vi "Review Modules Dialog.vi"(8 "error in":errorcluster, 11 "Potting Procedure in":refnum<class "Potting Procedure.lvclass">) -> (0 "error out":errorcluster, 2 "Canceled":bool, 3 "Potting Procedure out":refnum<class "Potting Procedure.lvclass">)   [LabVIEW 2011]
uses:
  Procedure Classes/Potting Procedure/Potting Procedure.lvclass
  Shared Components/Utils/Type Definitions/Fiducial with Source.ctl
  Shared Components/Vec3d Class/Vec3d Class.lvclass
  Procedure Classes/Potting Procedure/Type Definitions/Review Modules.ctl
  Procedure Classes/Potting Procedure/Type Definitions/Inspect Modules.ctl
  Shared Components/Utils/Type Definitions/Multi-Fiducial Image.ctl
  Shared Components/Utils/Type Definitions/Physical Image.ctl
  <vilib>/vision/Image Controls.llb/IMAQ Image.ctl
  Shared Components/Utils/Type Definitions/Fiducial Image.ctl
panel:
  in  "idx":i32
  out "idx_label":string="1/10"
  out "Current Module":cluster{"Chuck":i32, "Slot":i32}={"Chuck"=1, "Slot"=1}
  in  "Previous":bool
  in  "Next":bool
  in  "Tab Control":enum32{"Bond Pads", "TBM", "Address Pads & HV"}(tab)
  out "BBM-R":cluster{"X":dbl, "Y":dbl}[](graph)
  out "BBM-L":cluster{"X":dbl, "Y":dbl}[](graph)
  out "HDI-R":cluster{"X":dbl, "Y":dbl}[](graph)
  out "HDI-L":cluster{"X":dbl, "Y":dbl}[](graph)
  out "BBM BR":T1(plugin-control)
  out "BBM BL":T1(plugin-control)
  out "BBM TR":T1(plugin-control)
  out "BBM TL":T1(plugin-control)
  out "HDI BR":T1(plugin-control)
  out "HDI BL":T1(plugin-control)
  out "HDI TR":T1(plugin-control)
  out "HDI TL":T1(plugin-control)
  out "TBM-HDI":T1(plugin-control)
  out "TBM-TBM":T1(plugin-control)
  out "addr":T1(plugin-control) caption="Address Pads"
  out "HV-HDI":T1(plugin-control)
  out "HV-BBM":T1(plugin-control)
  in  "OK Button":bool
  in  "Cancel Button":bool
  # "Click on images to correct fiducial positions.\nAll error fiducials must be corrected before continuing."
  # "Pattern Recognition"
  # "Error"
  # "User Defined"
  # "Default"
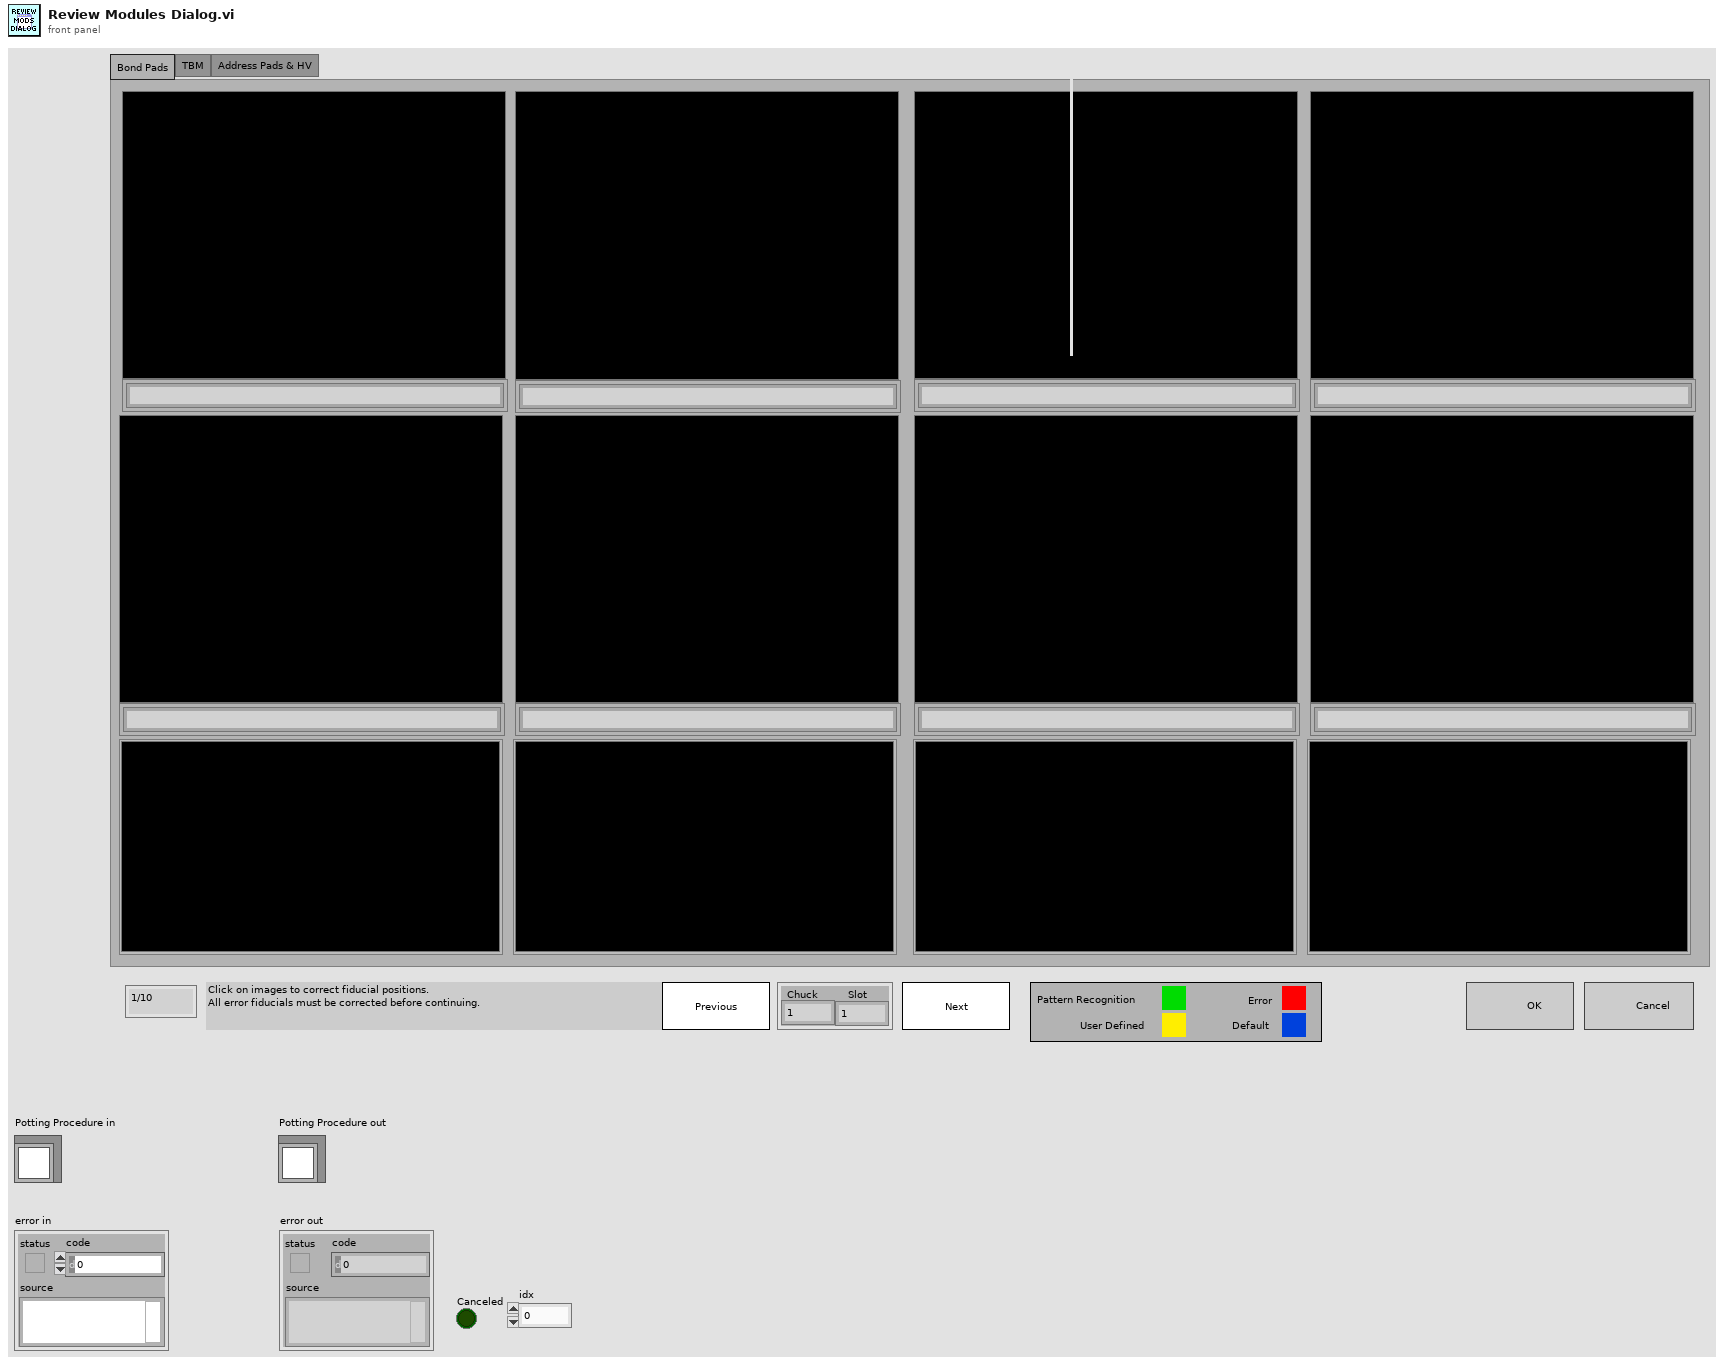
[diagram p1: front panel]
types:
  T1 = typedef "IMAQ Image.ctl" = refnum<image>
  T2 = typedef "Inspect Modules.ctl" = cluster{"Has Been Run?":bool, "Module Positions":cluster{"TBM-TBM":T3, "TBM-HDI":T3, "Address Pads":T3, "HDI Bond Pad References":T6[], "BBM Bond Pad References":T6[], "HV-HDI":T6, "HV-BBM":T6, "Chuck":i32, "Slot":i32}[]}
  T3 = typedef "Multi-Fiducial Image.ctl" = cluster{"Fiducial Image":T4, "Fiducials":cluster{"Selected Fiducial":T5, "fiducial name":string}[]}
  T4 = typedef "Physical Image.ctl" = cluster{"Image Position":refnum<class "Vec3d Class.lvclass">, "Image Reference":T1, "Field of View":cluster{"x(mm)":dbl, "y(mm)":dbl}}
  T5 = typedef "Fiducial with Source.ctl" = cluster{"Fiducial Image Coordinate":refnum<class "Vec3d Class.lvclass">, "Fiducial Source":enum16{"Pattern Recognition", "User", "Error", "Default"}}
  T6 = typedef "Fiducial Image.ctl" = cluster{"Fiducial Image":T4, "Selected Fiducial":T5, "fiducial name":string}
  T7 = cluster{"TBM-TBM":T3, "TBM-HDI":T3, "Address Pads":T3, "HDI Bond Pad References":T6[], "BBM Bond Pad References":T6[], "HV-HDI":T6, "HV-BBM":T6, "Chuck":i32, "Slot":i32}[]
  T8 = enum16{"Pattern Recognition", "User", "Error", "Default"}
  T9 = typedef "LVPoint32TypeDef.ctl" = cluster{"Horizontal":i32, "Vertical":i32}
  T10 = cluster{"TBM-TBM":T3, "TBM-HDI":T3, "Address Pads":T3, "HDI Bond Pad References":T6[], "BBM Bond Pad References":T6[], "HV-HDI":T6, "HV-BBM":T6, "Chuck":i32, "Slot":i32}
  T11 = cluster{"Selected Fiducial":T5, "fiducial name":string}[]
  T12 = cluster{"Selected Fiducial":T5, "fiducial name":string}
  T13 = typedef "eventvkey.ctl" = enum16{"ASCII", "Enter", "Return", "Shift", "Ctrl", "Alt", "Cmd", "Opt", "Caps", "NumLock", "Clear", "Break", "Up", "Down", "Left", "Right", "Insert", "Delete", "Home", "End", "PageUp", "PageDown", "Escape", "Help", "Pause", "ScrollLock", "F1", "F2", "F3", "F4", "F5", "F6", "F7", "F8", "F9", "F10", "F11", "F12", "F13", "F14", "F15", "F16", "F17", "F18", "F19", "F20", "F21", "F22", "F23", "F24", "Play", "VolumeUp", "VolumeDown", "Mute", "Two Byte Char"}
  T14 = typedef "Review Modules.ctl" = cluster{"Has Been Run?":bool}
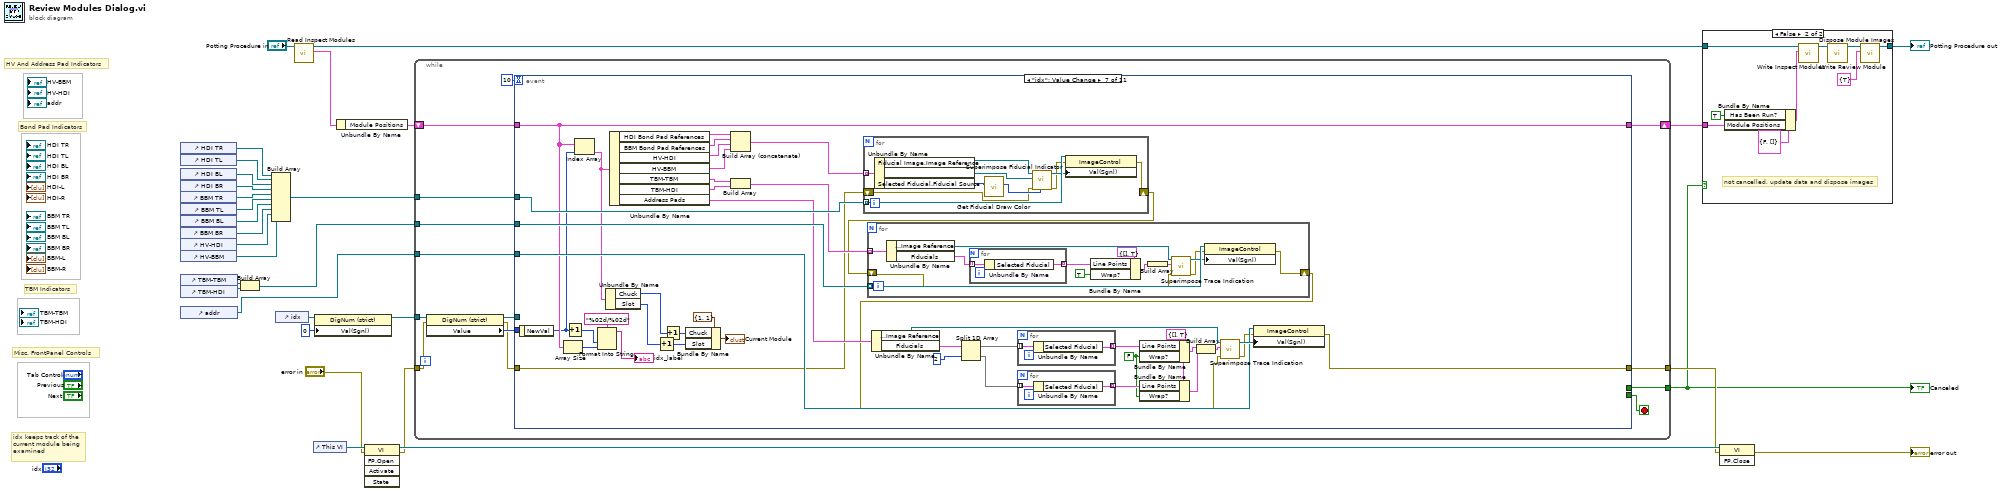
[diagram p0: block diagram]
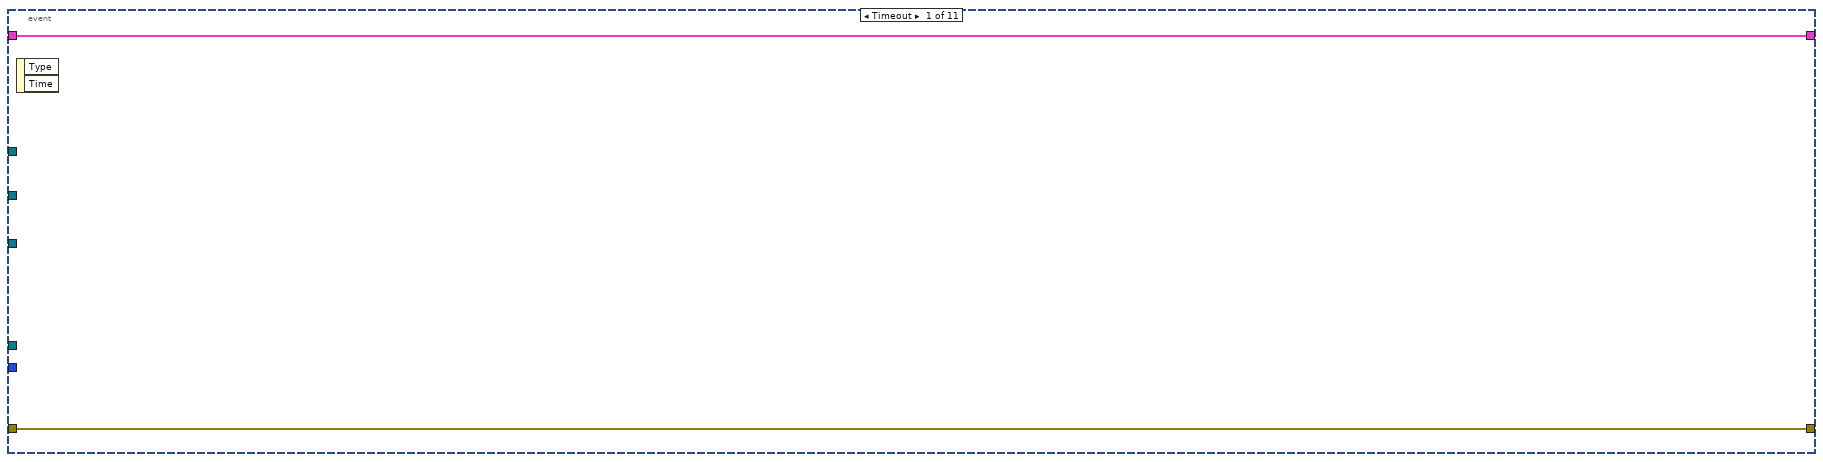
[diagram p3: hidden frame]
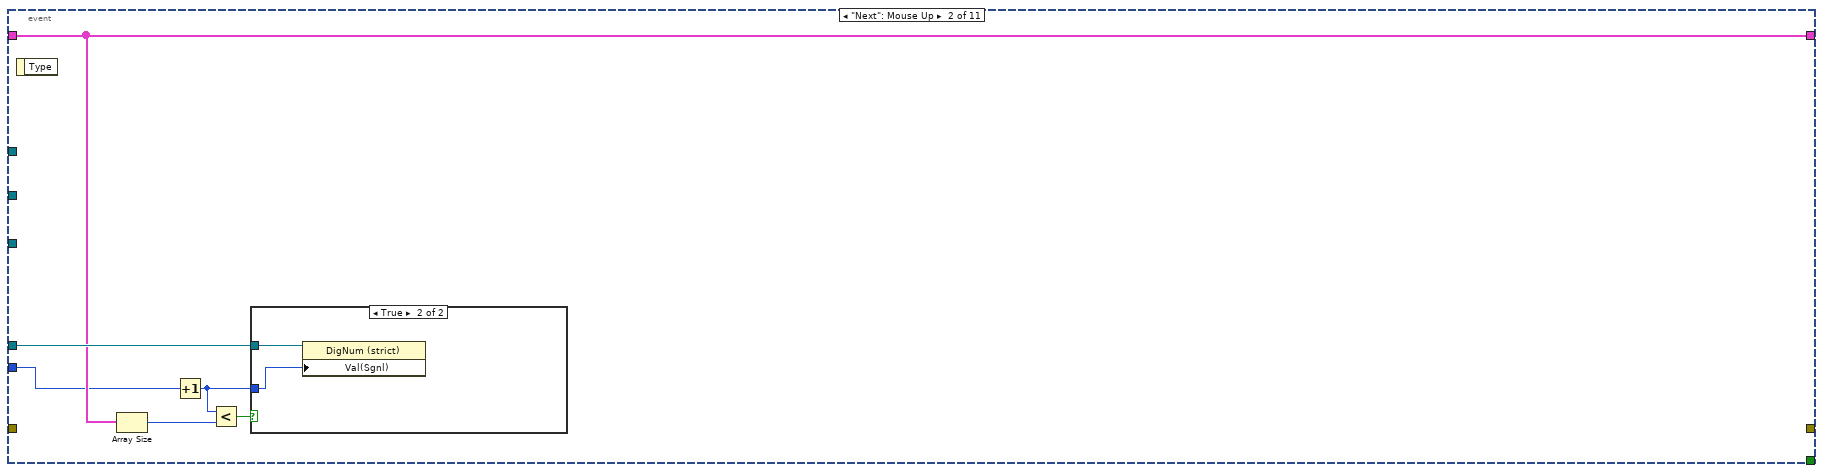
[diagram p4: hidden frame]
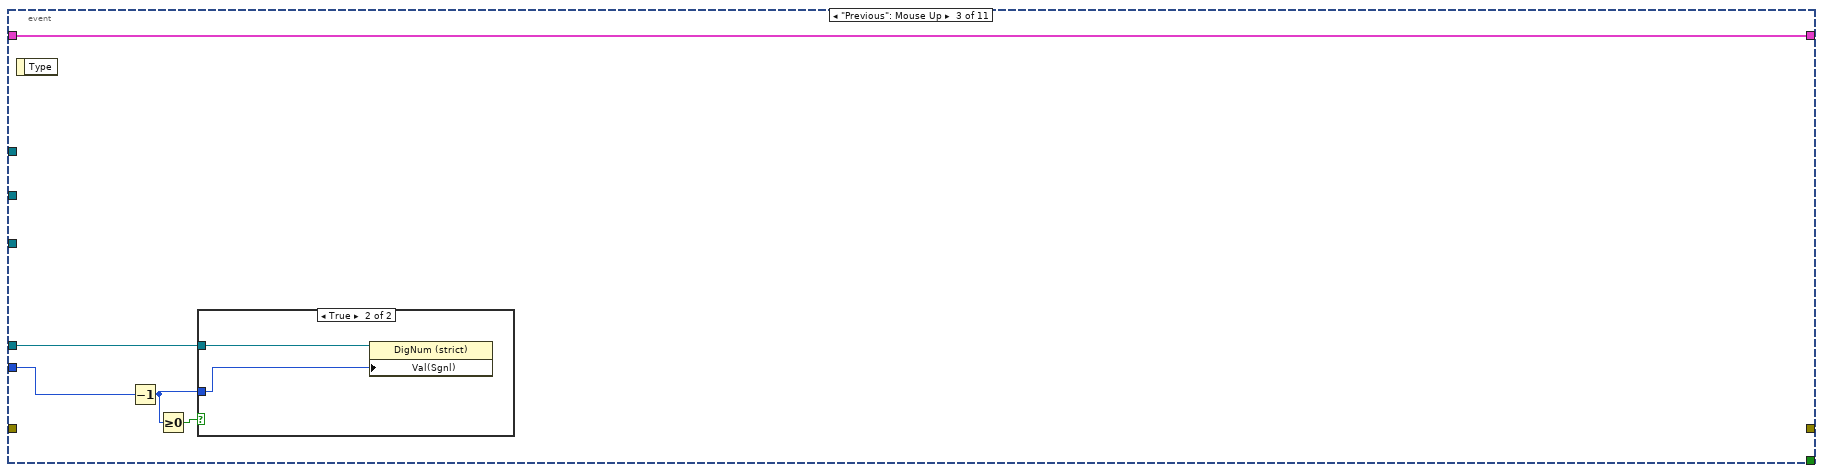
[diagram p6: hidden frame]
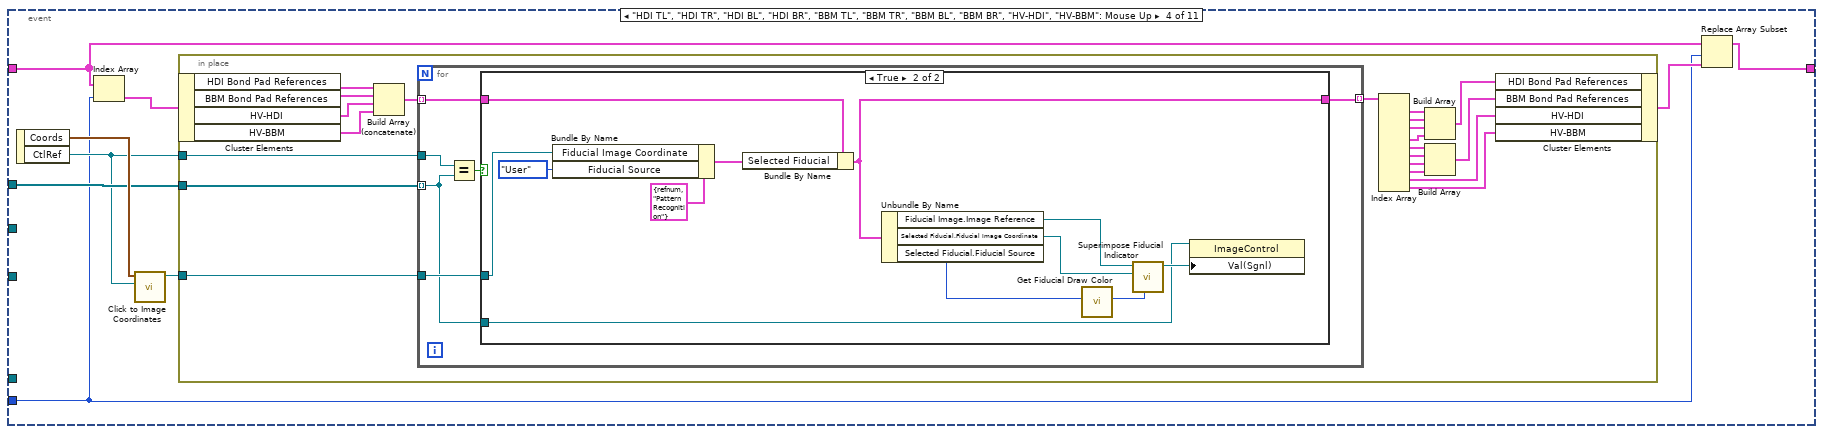
[diagram p8: hidden frame]
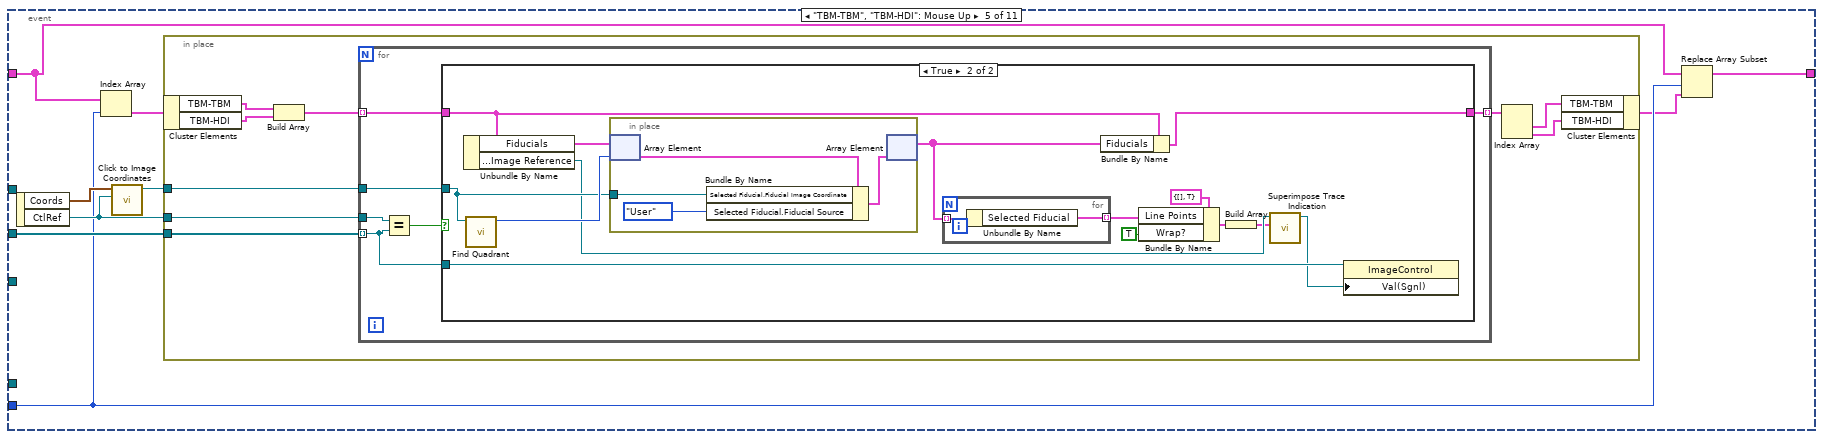
[diagram p10: hidden frame]
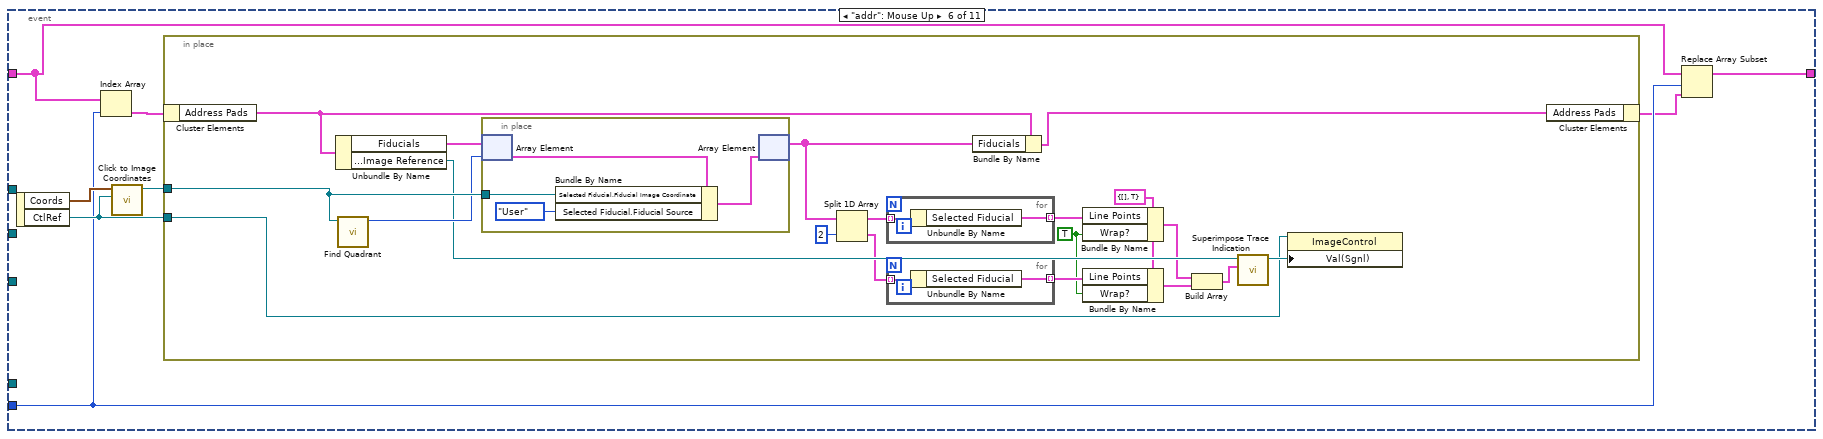
[diagram p12: hidden frame]
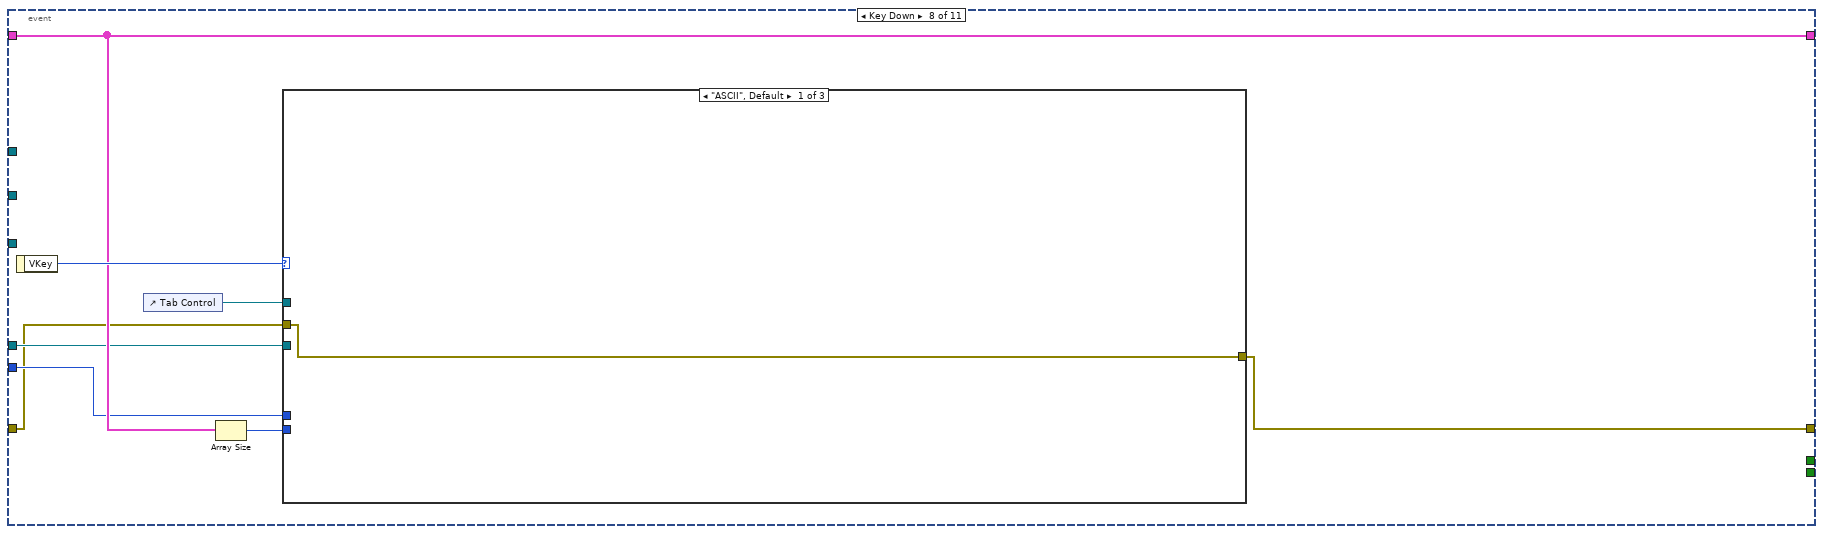
[diagram p13: hidden frame]
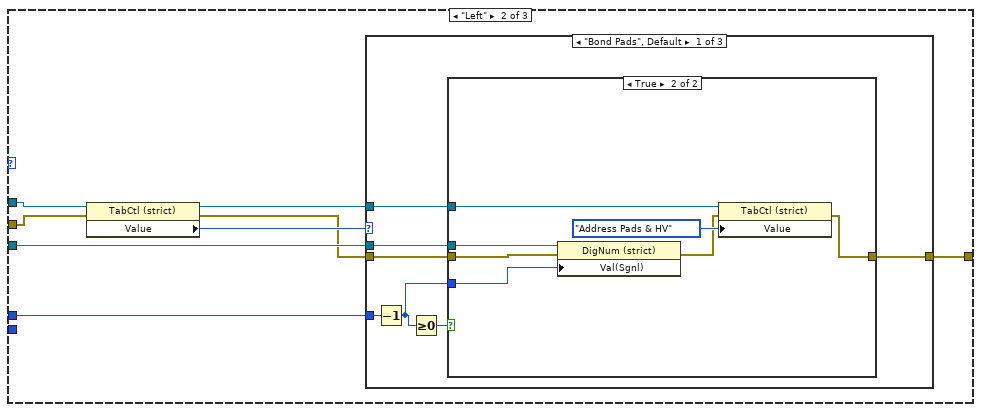
[diagram p14: hidden frame]
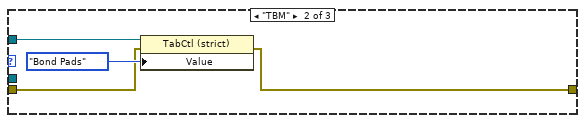
[diagram p16: hidden frame]
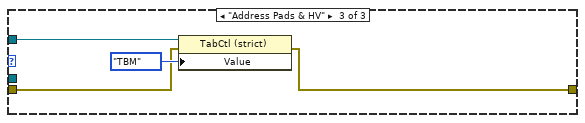
[diagram p17: hidden frame]
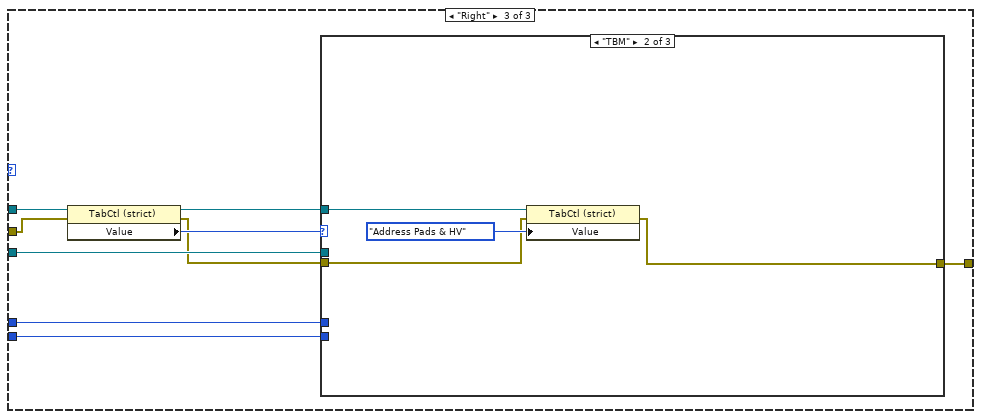
[diagram p18: hidden frame]
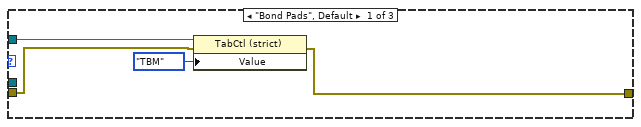
[diagram p19: hidden frame]
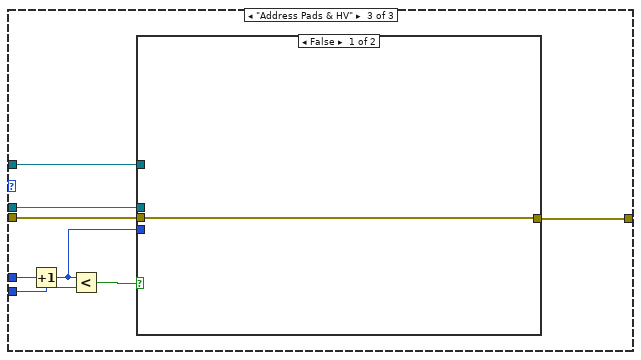
[diagram p20: hidden frame]
diagram:
  # "idx keeps track of the\ncurrent module being\nexamined"
  # "Misc. FrontPanel Controls"
  # "TBM Indicators"
  # "HV And Address Pad Indicators"
  # "Bond Pad Indicators"
  n1 = control-ref of="HDI TR"() -> (w22:refnum<vi>)
  n2 = control-ref of="HDI TL"() -> (w21:refnum<vi>)
  n3 = control-ref of="HDI BL"() -> (w20:refnum<vi>)
  n4 = control-ref of="HDI BR"() -> (w19:refnum<vi>)
  n5 = control-ref of="BBM TR"() -> (w18:refnum<vi>)
  n6 = control-ref of="BBM TL"() -> (w17:refnum<vi>)
  n7 = control-ref of="BBM BL"() -> (w16:refnum<vi>)
  n8 = control-ref of="BBM BR"() -> (w15:refnum<vi>)
  n9 = control-ref of="HV-HDI"() -> (w10:refnum<vi>)
  n10 = control-ref of="HV-BBM"() -> (w9:refnum<vi>)
  n11 = control-ref of="TBM-TBM"() -> (w13:refnum<vi>)
  n12 = control-ref of="TBM-HDI"() -> (w12:refnum<vi>)
  n13 = control-ref of="addr"() -> (w8:refnum<vi>)
  n14 = Build Array(w13, w12) -> (w11:refnum<vi>[])
  n15 = Build Array(w22, w21, w20, w19, w18, w17, w16, w15, w10, w9) -> (w14:refnum<vi>[])
  n16 = control-ref of="idx"() -> (w7:refnum<vi>)
  n17 = call-dynamic "Read Inspect Modules.vi"("Potting Procedure in"="Potting Procedure in") -> ("Inspect Modules"=w24:T2, "Potting Procedure out"=w2:refnum<class "Potting Procedure.lvclass">)  [unwired: 8 in, 1 out]
  n18 = control-ref of="This VI"() -> (w31:refnum<vi>)
  n19 = property class="DigNum (strict)"(reference=w7, "Val(Sgnl)"=0 ("Value (Signaling)")) -> (reference out=w6:refnum<vi>)  [unwired: 1 in, 1 out]
  n20 = Unbundle By Name(w24) -> ("Module Positions"=w23:T7)
  n21 = invoke class="VI" method="FP.Open"(reference=w31, error in="error in") -> (reference out=w30:refnum<vi>, error out=w27:errorcluster)  [unwired: 3 in, 3 out]
  n22 = while {
    tunnel: [w42] -> w4
    tunnel: w27 -> [w35]
    tunnel: [w43] -> w26
    shift-right: [w40] -> w3
    shift-left: w23 -> [w41]
    tunnel: w6 -> [w38]
    tunnel: w14 -> [w39]
    tunnel: w11 -> [w33]
    tunnel: w8 -> [w32]
    stop <- w44 stop-if-true
    n23 = property class="DigNum (strict)"(reference=w38, error in=w35) -> (reference out=w37:refnum<vi>, error out=w34:errorcluster, "Value"=w36:i32)
    n24 = event shown="[6] \"idx\": Value Change" {
      selector: _ -> [_ _ _ _ _ _ _ _ _ _ _]
      dyn-events: _ -> [_ _ _ _ _ _ _ _ _ _ _]
      timeout: 10 -> [_ _ _ _ _ _ _ _ _ _ _]
      tunnel: [_ _ _ _ _ _ _ _ w338 w340 _] -> w44
      tunnel: [w47 _ _ _ _ _ w205 w264 w339 w342 w345] -> w43
      tunnel: w34 -> [w47 _ _ _ _ _ w209 w265 w339 w342 w345]
      tunnel: [_ _ _ _ _ _ _ _ w338 _ _] -> w42
      tunnel: w41 -> [w46 w49 w57 w66 w113 w158 w195 w269 w337 w341 w344]
      tunnel: [w46 w49 w57 w63 w112 w157 w195 w269 w337 w341 w344] -> w40
      tunnel: w37 -> [_ w51 w58 _ _ _ _ w266 _ _ _]
      tunnel: w39 -> [_ _ _ w69 _ _ w227 _ _ _ _]
      tunnel: w36 -> [_ w48 w56 w64 w115 w160 _ w267 _ _ _]
      tunnel: w33 -> [_ _ _ _ w118 _ w225 _ _ _ _]
      tunnel: w32 -> [_ _ _ _ _ _ w218 _ _ _ _]
      event Timeout {
        n25 = event-data() -> ()  [unwired: 1 in, 2 out]
      }
      event "Next": Mouse Up {
        n26 = event-data() -> ()  [unwired: 1 in, 1 out]
        n27 = Array Size(array=w49) -> (size(s)=w50:i32)
        n28 = Increment(x=w48) -> (x+1=w52:i32)
        n29 = Less?(x=w52, y=w50) -> (x < y?=w53:bool)
        n30 = case shown="True" w53 {
          tunnel: w52 -> [_ w54]
          tunnel: w51 -> [_ w55]
          frame False {
          }
          frame True {
            n31 = property class="DigNum (strict)"(reference=w55, "Val(Sgnl)"=w54) -> ()  [unwired: 1 in, 2 out]
          }
        }
      }
      event "Previous": Mouse Up {
        n32 = event-data() -> ()  [unwired: 1 in, 1 out]
        n33 = Decrement(x=w56) -> (x-1=w59:i32)
        n34 = Greater Or Equal To 0?(x=w59) -> (x >= 0?=w60:bool)
        n35 = case shown="True" w60 {
          tunnel: w59 -> [_ w61]
          tunnel: w58 -> [_ w62]
          frame False {
          }
          frame True {
            n36 = property class="DigNum (strict)"(reference=w62, "Val(Sgnl)"=w61) -> ()  [unwired: 1 in, 2 out]
          }
        }
      }
      event "HDI TL", "HDI TR", "HDI BL", "HDI BR", "BBM TL", "BBM TR", "BBM BL", "BBM BR", "HV-HDI", "HV-BBM": Mouse Up {
        n37 = event-data() -> ("Coords"=w71:T9, "CtlRef"=w68:refnum<vi>)  [unwired: 1 in]
        n38 = Index Array(array=w66, index=w64) -> (element=w67:T10)
        n39 = call "Click to Image Coordinates.vi"("Display Reference"=w68, "Coords"=w71) -> ("Image Coordinates"=w70:refnum<class "Vec3d Class.lvclass">)  [unwired: 8 in, 1 out]
        n40 = in-place {
          in-place-border: w70 -> [w91]
          in-place-border: w69 -> [w90]
          in-place-border: w68 -> [w89]
          n41 = in-place-cluster #1(w67) -> ("HDI Bond Pad References"=w88:T6[], "BBM Bond Pad References"=w87:T6[], "HV-HDI"=w86:T6, "HV-BBM"=w85:T6)
          n42 = Build Array (concatenate)(w88, w87, w86, w85) -> (w92:T6[])
          n43 = for {
            tunnel: w92 -> [w95] mode=indexing
            tunnel: w91 -> [w96]
            tunnel: w90 -> [w94] mode=indexing
            tunnel: w89 -> [w98]
            tunnel: [w93] -> w84 mode=indexing
            n44 = Equal?(x=w98, y=w94) -> (x = y?=w97:bool)
            n45 = case shown="True" w97 {
              tunnel: w96 -> [_ w109]
              tunnel: w95 -> [w99 w111]
              tunnel: [w99 w106] -> w93
              tunnel: w94 -> [_ w102]
              frame False {
              }
              frame True {
                n46 = Bundle By Name(cluster=T5 {"Fiducial Image Coordinate"=refnum, "Fiducial Source"=enum."Pattern Recognition"} ("Selected Fiducial"), "Fiducial Image Coordinate"=w109, "Fiducial Source"=T8."User") -> (w107:T5)
                n47 = Bundle By Name(cluster=w111, "Selected Fiducial"=w107) -> (w106:T6)
                n48 = Unbundle By Name(w106) -> ("Fiducial Image.Image Reference"=w103:T1, "Selected Fiducial.Fiducial Image Coordinate"=w104:refnum<class "Vec3d Class.lvclass">, "Selected Fiducial.Fiducial Source"=w101:T8)
                n49 = call "Get Fiducial Draw Color.vi"("Fiducial Source"=w101) -> ("Grid Line Color"=w100:u32)  [unwired: 10 in]
                n50 = call "Superimpose Fiducial Indicator.vi"("Marker Color"=w100, "Fiducial Image Coordinates"=w104, "Image In"=w103) -> ("Image Out"=w105:T1)  [unwired: 7 in, 1 out]
                n51 = property class="ImageControl"(reference=w102, "Val(Sgnl)"=w105) -> ()  [unwired: 1 in, 2 out]
              }
            }
          }
          n52 = Index Array(array=w84) -> (element #1=w83:T6, element #2=w82:T6, element #3=w81:T6, element #4=w80:T6, element #5=w78:T6, element #6=w77:T6, element #7=w76:T6, element #8=w75:T6, element #9=w73:T6, element #10=w72:T6)  [unwired: 10 in]
          n53 = Build Array(w83, w82, w81, w80) -> (w79:T6[])
          n54 = Build Array(w78, w77, w76, w75) -> (w74:T6[])
          n55 = in-place-cluster #1("HDI Bond Pad References"=w79, "BBM Bond Pad References"=w74, "HV-HDI"=w73, "HV-BBM"=w72) -> (w65:T10)
        }
        n56 = Replace Array Subset(array=w66, new element=w65, index=w64) -> (w63:T7)
      }
      event "TBM-TBM", "TBM-HDI": Mouse Up {
        n57 = event-data() -> ("Coords"=w120:T9, "CtlRef"=w119:refnum<vi>)  [unwired: 1 in]
        n58 = Index Array(array=w113, index=w115) -> (element=w116:T10)
        n59 = call "Click to Image Coordinates.vi"("Display Reference"=w119, "Coords"=w120) -> ("Image Coordinates"=w117:refnum<class "Vec3d Class.lvclass">)  [unwired: 8 in, 1 out]
        n60 = in-place {
          in-place-border: w119 -> [w128]
          in-place-border: w118 -> [w127]
          in-place-border: w117 -> [w126]
          n61 = in-place-cluster #2(w116) -> ("TBM-TBM"=w125:T3, "TBM-HDI"=w124:T3)
          n62 = Build Array(w125, w124) -> (w129:T3[])
          n63 = for {
            tunnel: w129 -> [w133] mode=indexing
            tunnel: w128 -> [w135]
            tunnel: w127 -> [w131] mode=indexing
            tunnel: w126 -> [w132]
            tunnel: [w130] -> w123 mode=indexing
            n64 = Equal?(x=w135, y=w131) -> (x = y?=w134:bool)
            n65 = case shown="True" w134 {
              tunnel: w133 -> [w136 w147]
              tunnel: w132 -> [_ w148]
              tunnel: [w136 w146] -> w130
              tunnel: w131 -> [_ w138]
              frame False {
              }
              frame True {
                n66 = Unbundle By Name(w147) -> ("Fiducials"=w150:T11, "Fiducial Image.Image Reference"=w142:T1)
                n67 = call "Find Quadrant.vi"("Image Coordinate"=w148) -> ("Quadrant"=w149:i32)  [unwired: 10 in]
                n68 = in-place {
                  in-place-border: w148 -> [w154]
                  n69 = in-place-array #3(w150, w149) -> (w156:T12)
                  n70 = Bundle By Name(cluster=w156, "Selected Fiducial.Fiducial Image Coordinate"=w154, "Selected Fiducial.Fiducial Source"=T8."User") -> (w155:T12)
                  n71 = in-place-array #3(w155) -> (w145:T11)  [unwired: 1 out]
                }
                n72 = for {
                  tunnel: w145 -> [w152] mode=indexing
                  tunnel: [w151] -> w141 mode=indexing
                  n73 = Unbundle By Name(w152) -> ("Selected Fiducial"=w151:T5)
                }
                n74 = Bundle By Name(cluster=w147, "Fiducials"=w145) -> (w146:T3)
                n75 = Bundle By Name(cluster=cluster{"Line Points":T5[], "Wrap?":bool} {"Line Points"=[], "Wrap?"=TRUE} ("Line Group"), "Line Points"=w141, "Wrap?"=TRUE) -> (w144:cluster{"Line Points":T5[], "Wrap?":bool})
                n76 = Build Array(w144) -> (w139:cluster{"Line Points":T5[], "Wrap?":bool}[])
                n77 = call "Superimpose Trace Indication.vi"("Line Data"=w139, "Image In"=w142) -> ("Image Out"=w137:T1)  [unwired: 8 in, 1 out]
                n78 = property class="ImageControl"(reference=w138, "Val(Sgnl)"=w137) -> ()  [unwired: 1 in, 2 out]
              }
            }
          }
          n79 = Index Array(array=w123) -> (element #1=w122:T3, element #2=w121:T3)  [unwired: 2 in]
          n80 = in-place-cluster #2("TBM-TBM"=w122, "TBM-HDI"=w121) -> (w114:T10)
        }
        n81 = Replace Array Subset(array=w113, new element=w114, index=w115) -> (w112:T7)
      }
      event "addr": Mouse Up {
        n82 = event-data() -> ("Coords"=w164:T9, "CtlRef"=w163:refnum<vi>)  [unwired: 1 in]
        n83 = Index Array(array=w158, index=w160) -> (element=w161:T10)
        n84 = call "Click to Image Coordinates.vi"("Display Reference"=w163, "Coords"=w164) -> ("Image Coordinates"=w162:refnum<class "Vec3d Class.lvclass">)  [unwired: 8 in, 1 out]
        n85 = in-place {
          in-place-border: w163 -> [w174]
          in-place-border: w162 -> [w183]
          w165 = cluster{"Line Points":T5[], "Wrap?":bool} {"Line Points"=[], "Wrap?"=TRUE} ("Line Group")
          w168 = TRUE ("Wrap?")
          n86 = in-place-cluster #4(w161) -> ("Address Pads"=w181:T3)
          n87 = Unbundle By Name(w181) -> ("Fiducials"=w180:T11, "Fiducial Image.Image Reference"=w178:T1)
          n88 = call "Find Quadrant.vi"("Image Coordinate"=w183) -> ("Quadrant"=w179:i32)  [unwired: 10 in]
          n89 = in-place {
            in-place-border: w183 -> [w189]
            n90 = in-place-array #5(w180, w179) -> (w191:T12)
            n91 = Bundle By Name(cluster=w191, "Selected Fiducial.Fiducial Image Coordinate"=w189, "Selected Fiducial.Fiducial Source"=T8."User") -> (w190:T12)
            n92 = in-place-array #5(w190) -> (w172:T11)  [unwired: 1 out]
          }
          n93 = Split 1D Array(array=w172, index=2) -> (first subarray=w171:T11, second subarray=w170:T11)
          n94 = for {
            tunnel: [w186] -> _ mode=indexing
            tunnel: [w187] -> w177 mode=indexing
            tunnel: w171 -> [w186] mode=indexing
            n95 = Unbundle By Name(w186) -> ("Selected Fiducial"=w187:T5)
          }
          n96 = for {
            tunnel: w170 -> [w185] mode=indexing
            tunnel: [w184] -> w173 mode=indexing
            n97 = Unbundle By Name(w185) -> ("Selected Fiducial"=w184:T5)
          }
          n98 = Bundle By Name(cluster=w181, "Fiducials"=w172) -> (w182:T3)
          n99 = Bundle By Name(cluster=w165, "Line Points"=w177, "Wrap?"=w168) -> (w167:cluster{"Line Points":T5[], "Wrap?":bool})
          n100 = Bundle By Name(cluster=w165, "Line Points"=w173, "Wrap?"=w168) -> (w166:cluster{"Line Points":T5[], "Wrap?":bool})
          n101 = Build Array(w167, w166) -> (w176:cluster{"Line Points":T5[], "Wrap?":bool}[])
          n102 = call "Superimpose Trace Indication.vi"("Line Data"=w176, "Image In"=w178) -> ("Image Out"=w175:T1)  [unwired: 8 in, 1 out]
          n103 = property class="ImageControl"(reference=w174, "Val(Sgnl)"=w175) -> ()  [unwired: 1 in, 2 out]
          n104 = in-place-cluster #4("Address Pads"=w182) -> (w159:T10)
        }
        n105 = Replace Array Subset(array=w158, new element=w159, index=w160) -> (w157:T7)
      }
      event "idx": Value Change {
        w212 = FALSE ("Wrap?")
        w211 = cluster{"Line Points":T5[], "Wrap?":bool} {"Line Points"=[], "Wrap?"=TRUE} ("Line Group")
        n106 = event-data() -> ("NewVal"=w194:i32)  [unwired: 1 in]
        n107 = Array Size(array=w195) -> (size(s)=w201:i32)
        n108 = Increment(x=w194) -> (x+1=w202:i32)
        n109 = Index Array(array=w195, index=w194) -> (element=w196:T10)
        n110 = Format Into String(format string="%02d/%02d", w202, w201) -> (resulting string=→"idx_label":string)  [unwired: 2 in, 1 out]
        n111 = Unbundle By Name(w196) -> ("Chuck"=w193:i32, "Slot"=w192:i32)
        n112 = Unbundle By Name(w196) -> ("HDI Bond Pad References"=w234:T6[], "BBM Bond Pad References"=w233:T6[], "HV-HDI"=w232:T6, "HV-BBM"=w231:T6, "TBM-TBM"=w230:T3, "TBM-HDI"=w229:T3, "Address Pads"=w219:T3)
        n113 = Increment(x=w192) -> (x+1=w200:i32)
        n114 = Increment(x=w193) -> (x+1=w199:i32)
        n115 = Bundle By Name(cluster=cluster{"Chuck":i32, "Slot":i32} {"Chuck"=1, "Slot"=1} ("Current Module"), "Chuck"=w199, "Slot"=w200) -> (→"Current Module":cluster{"Chuck":i32, "Slot":i32})
        n116 = Build Array (concatenate)(w234, w233, w232, w231) -> (w228:T6[])
        n117 = Build Array(w230, w229) -> (w226:T3[])
        n118 = for {
          tunnel: w227 -> [w258] mode=indexing
          tunnel: w228 -> [w263] mode=indexing
          shift-right: [w254] -> w208
          shift-left: w209 -> [w256]
          n119 = Unbundle By Name(w263) -> ("Fiducial Image.Image Reference"=w262:T1, "Selected Fiducial.Fiducial Image Coordinate"=w261:refnum<class "Vec3d Class.lvclass">, "Selected Fiducial.Fiducial Source"=w260:T8)
          n120 = call "Get Fiducial Draw Color.vi"("Fiducial Source"=w260) -> ("Grid Line Color"=w259:u32)  [unwired: 10 in]
          n121 = call "Superimpose Fiducial Indicator.vi"("Marker Color"=w259, "error in"=w256, "Fiducial Image Coordinates"=w261, "Image In"=w262) -> ("error out"=w255:errorcluster, "Image Out"=w257:T1)  [unwired: 6 in]
          n122 = property class="ImageControl"(reference=w258, error in=w255, "Val(Sgnl)"=w257) -> (error out=w254:errorcluster)  [unwired: 1 out]
        }
        n123 = for {
          tunnel: w225 -> [w249] mode=indexing
          tunnel: w226 -> [w251] mode=indexing
          shift-right: [w239] -> w207
          shift-left: w208 -> [w241]
          n124 = Unbundle By Name(w251) -> ("Fiducial Image.Image Reference"=w250:T1, "Fiducials"=w247:T11)
          n125 = for {
            tunnel: w247 -> [w253] mode=indexing
            tunnel: [w252] -> w245 mode=indexing
            n126 = Unbundle By Name(w253) -> ("Selected Fiducial"=w252:T5)
          }
          n127 = Bundle By Name(cluster=cluster{"Line Points":T5[], "Wrap?":bool} {"Line Points"=[], "Wrap?"=TRUE} ("Line Group"), "Line Points"=w245, "Wrap?"=TRUE) -> (w243:cluster{"Line Points":T5[], "Wrap?":bool})
          n128 = Build Array(w243) -> (w242:cluster{"Line Points":T5[], "Wrap?":bool}[])
          n129 = call "Superimpose Trace Indication.vi"("error in"=w241, "Line Data"=w242, "Image In"=w250) -> ("error out"=w240:errorcluster, "Image Out"=w248:T1)  [unwired: 7 in]
          n130 = property class="ImageControl"(reference=w249, error in=w240, "Val(Sgnl)"=w248) -> (error out=w239:errorcluster)  [unwired: 1 out]
        }
        n131 = Unbundle By Name(w219) -> ("Fiducial Image.Image Reference"=w224:T1, "Fiducials"=w217:T11)
        n132 = Split 1D Array(array=w217, index=2) -> (first subarray=w215:T11, second subarray=w214:T11)
        n133 = for {
          tunnel: w215 -> [w238] mode=indexing
          tunnel: [w237] -> w222 mode=indexing
          n134 = Unbundle By Name(w238) -> ("Selected Fiducial"=w237:T5)
        }
        n135 = for {
          tunnel: w214 -> [w236] mode=indexing
          tunnel: [w235] -> w213 mode=indexing
          n136 = Unbundle By Name(w236) -> ("Selected Fiducial"=w235:T5)
        }
        n137 = Bundle By Name(cluster=w211, "Line Points"=w222, "Wrap?"=w212) -> (w221:cluster{"Line Points":T5[], "Wrap?":bool})
        n138 = Bundle By Name(cluster=w211, "Line Points"=w213, "Wrap?"=w212) -> (w210:cluster{"Line Points":T5[], "Wrap?":bool})
        n139 = Build Array(w221, w210) -> (w220:cluster{"Line Points":T5[], "Wrap?":bool}[])
        n140 = call "Superimpose Trace Indication.vi"("error in"=w207, "Line Data"=w220, "Image In"=w224) -> ("error out"=w206:errorcluster, "Image Out"=w223:T1)  [unwired: 7 in]
        n141 = property class="ImageControl"(reference=w218, error in=w206, "Val(Sgnl)"=w223) -> (error out=w205:errorcluster)  [unwired: 1 out]
      }
      event Key Down {
        n142 = event-data() -> ("VKey"=w271:T13)  [unwired: 1 in]
        n143 = control-ref of="Tab Control"() -> (w270:refnum<vi>)
        n144 = Array Size(array=w269) -> (size(s)=w268:i32)
        n145 = case shown="\"ASCII\", Default" w271 {
          tunnel: w270 -> [_ w276 w312]
          tunnel: w268 -> [_ _ w308]
          tunnel: w267 -> [_ w277 w307]
          tunnel: w266 -> [_ w278 w309]
          tunnel: w265 -> [w272 w275 w306]
          tunnel: [w272 w273 w304] -> w264
          frame "ASCII", Default {
          }
          frame "Left" {
            n146 = property class="TabCtl (strict)"(reference=w276, error in=w275) -> (reference out=w279:refnum<vi>, error out=w274:errorcluster, "Value"=w280:enum32{"Bond Pads", "TBM", "Address Pads & HV"})
            n147 = case shown="\"Bond Pads\", Default" w280 {
              tunnel: w279 -> [w287 w299 w302]
              tunnel: w278 -> [w286 _ _]
              tunnel: w277 -> [w285 _ _]
              tunnel: w274 -> [w282 w297 w301]
              tunnel: [w281 w296 w300] -> w273
              frame "Bond Pads", Default {
                n148 = Decrement(x=w285) -> (x-1=w283:i32)
                n149 = Greater Or Equal To 0?(x=w283) -> (x >= 0?=w284:bool)
                n150 = case shown="True" w284 {
                  tunnel: w286 -> [_ w295]
                  tunnel: w287 -> [_ w294]
                  tunnel: w283 -> [_ w292]
                  tunnel: w282 -> [w288 w291]
                  tunnel: [w288 w289] -> w281
                  frame False {
                  }
                  frame True {
                    n151 = property class="DigNum (strict)"(reference=w295, error in=w291, "Val(Sgnl)"=w292) -> (error out=w290:errorcluster)  [unwired: 1 out]
                    n152 = property class="TabCtl (strict)"(reference=w294, error in=w290, "Value"=enum32{"Bond Pads", "TBM", "Address Pads & HV"}."Address Pads & HV") -> (error out=w289:errorcluster)  [unwired: 1 out]
                  }
                }
              }
              frame "TBM" {
                n153 = property class="TabCtl (strict)"(reference=w299, error in=w297, "Value"=enum32{"Bond Pads", "TBM", "Address Pads & HV"}."Bond Pads") -> (error out=w296:errorcluster)  [unwired: 1 out]
              }
              frame "Address Pads & HV" {
                n154 = property class="TabCtl (strict)"(reference=w302, error in=w301, "Value"=enum32{"Bond Pads", "TBM", "Address Pads & HV"}."TBM") -> (error out=w300:errorcluster)  [unwired: 1 out]
              }
            }
          }
          frame "Right" {
            n155 = property class="TabCtl (strict)"(reference=w312, error in=w306) -> (reference out=w310:refnum<vi>, error out=w305:errorcluster, "Value"=w311:enum32{"Bond Pads", "TBM", "Address Pads & HV"})
            n156 = case shown="\"TBM\"" w311 {
              tunnel: w310 -> [w315 w320 w323]
              tunnel: w309 -> [_ _ w325]
              tunnel: w308 -> [_ _ w327]
              tunnel: w307 -> [_ _ w328]
              tunnel: w305 -> [w314 w318 w322]
              tunnel: [w313 w317 w321] -> w304
              frame "Bond Pads", Default {
                n157 = property class="TabCtl (strict)"(reference=w315, error in=w314, "Value"=enum32{"Bond Pads", "TBM", "Address Pads & HV"}."TBM") -> (error out=w313:errorcluster)  [unwired: 1 out]
              }
              frame "TBM" {
                n158 = property class="TabCtl (strict)"(reference=w320, error in=w318, "Value"=enum32{"Bond Pads", "TBM", "Address Pads & HV"}."Address Pads & HV") -> (error out=w317:errorcluster)  [unwired: 1 out]
              }
              frame "Address Pads & HV" {
                n159 = Increment(x=w328) -> (x+1=w324:i32)
                n160 = Less?(x=w324, y=w327) -> (x < y?=w326:bool)
                n161 = case shown="False" w326 {
                  tunnel: w325 -> [_ w336]
                  tunnel: w324 -> [_ w335]
                  tunnel: w323 -> [_ w334]
                  tunnel: w322 -> [w329 w332]
                  tunnel: [w329 w330] -> w321
                  frame False {
                  }
                  frame True {
                    n162 = property class="DigNum (strict)"(reference=w336, error in=w332, "Val(Sgnl)"=w335) -> (error out=w331:errorcluster)  [unwired: 1 out]
                    n163 = property class="TabCtl (strict)"(reference=w334, error in=w331, "Value"=enum32{"Bond Pads", "TBM", "Address Pads & HV"}."Bond Pads") -> (error out=w330:errorcluster)  [unwired: 1 out]
                  }
                }
              }
            }
          }
        }
      }
      event "Cancel Button": Mouse Up {
        w338 = TRUE
        n164 = event-data() -> ()  [unwired: 1 in, 2 out]
      }
      event "OK Button": Mouse Up {
        # "Check that there are no\nError Fiducials"
        n165 = event-data() -> ()  [unwired: 1 in, 2 out]
        n166 = call "Verify Module Positions.vi"("Module Positions In"=w341) -> ("All Good"=w340:bool)  [unwired: 9 in, 1 out]
        n167 = case shown="False" w340 {
          frame False {
            n168 = One Button Dialog(message="Cannot Proceed with any \"Error\" markers.\nCorrect these before proceeding") -> ()  [unwired: 1 in, 1 out]
          }
          frame True {
          }
        }
      }
      event Panel Close? {
        # "This event disables the windows \"X\""
        n169 = event-data() -> ()  [unwired: 1 in, 3 out]
        n170 = event-data("Discard?"=FALSE) -> ()  [unwired: 1 in, 1 out]
      }
    }
  }
  "Canceled" <- w4
  n171 = case shown="False" w4 {
    tunnel: w3 -> [_ w354]
    tunnel: w2 -> [w347 w356]
    tunnel: [w347 w350] -> w1
    frame True {
      # "cancelled, do nothing"
    }
    frame False {
      # "not cancelled, update data and dispose images"
      n172 = Bundle By Name(cluster=T2 {"Has Been Run?"=FALSE, "Module Positions"=[]} ("Inspect Modules"), "Has Been Run?"=TRUE, "Module Positions"=w354) -> (w352:T2)
      n173 = call-dynamic "Write Inspect Modules.vi"("Inspect Modules"=w352, "Potting Procedure in"=w356) -> ("Potting Procedure out"=w349:refnum<class "Potting Procedure.lvclass">)  [unwired: 8 in, 1 out]
      n174 = call-dynamic "Dispose Module Images.vi"("Potting Procedure in"=w349) -> ("Potting Procedure out"=w348:refnum<class "Potting Procedure.lvclass">)  [unwired: 9 in, 1 out]
      n175 = call-dynamic "Write Review Module.vi"("Review Modules"=T14 {"Has Been Run?"=TRUE}, "Potting Procedure in"=w348) -> ("Potting Procedure out"=w350:refnum<class "Potting Procedure.lvclass">)  [unwired: 8 in, 1 out]
    }
  }
  "Potting Procedure out" <- w1
  n176 = invoke class="VI" method="FP.Close"(reference=w30, error in=w26) -> (error out=→"error out":errorcluster)  [unwired: 1 in, 2 out]
